vi "Strip String Ends.vi"(11 "String in":string) -> (3 "String out":string)   [LabVIEW 2021]
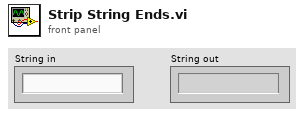
[diagram p1: front panel]
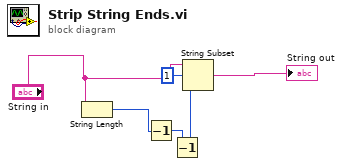
[diagram p0: block diagram]
diagram:
  n1 = String Length(string="String in") -> (length=w3:i32)
  n2 = Decrement(x=w3) -> (x-1=w4:i32)
  n3 = Decrement(x=w4) -> (x-1=w5:i32)
  n4 = String Subset(string="String in", offset (0)=1, length (rest)=w5) -> (substring=→"String out":string)
